vi "Atto DRY Interface start Sample Exchange.vi"(8 "error in (no error)":errorcluster) -> (0 "error out":errorcluster, 3 "function return":i32)   [LabVIEW 2016, in "attoDRYLib.lvlib"]
doc: "int32_t __cdecl AttoDRY_Interface_startSampleExchange(void);"
uses:
  <userlib>/attoDRYLib/attoDRYLib.lvlib
  <userlib>/attoDRYLib/attoDRYLib.dll
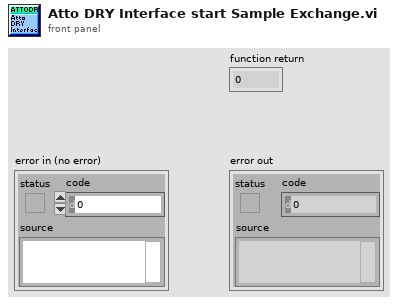
[diagram p1: front panel]
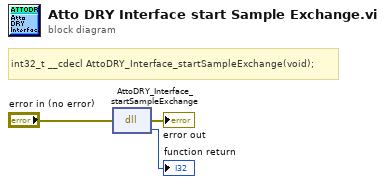
[diagram p0: block diagram]
diagram:
  # "int32_t __cdecl AttoDRY_Interface_startSampleExchange(void);"
  n1 = dll-call lib="C:/Program Files (x86)/National Instruments/LabVIEW 2016/user.lib/attoDRYLib/attoDRYLib.*" fn="AttoDRY_Interface_startSampleExchange"(error in="error in (no error)") -> (error out=→"error out":errorcluster, →"function return":i32)  [unwired: 2 in, 1 out]
